vi "Process.vi"(8 "error in":errorcluster, 11 "SynchIO":refnum<class "SynchIO.lvclass">) -> (0 "error out":errorcluster, 3 "SynchIO out":refnum<class "SynchIO.lvclass">)   [LabVIEW 2016, in "SynchIO.lvclass"]
doc: "---------------------------------------------------------------\nJKI State Machine Objects™\nhttp://jki.net/state-machine-objects/\nCopyright (C) 2005-2015, JKI <info@jki.net>\nALL RIGHTS RESERVEDJKI State Machine Objects (SMO) 1.0.0.5\nJKI - JKI\nCopyright (c) 2016, JKI"
uses:
  SynchIO.lvclass
  C:/Program Files (x86)/National Instruments/LabVIEW 2016/vi.lib/JKI/JKI SMO/SMO/SMO.lvclass
  <vilib>/JKI/JKI SMO/SMO/Typedefs/Parent Call--Enum.ctl
  <vilib>/JKI/JKI SMO/SMO/SMO.lvclass
panel:
  # "For instructions on how to use the JKI State Machine Objects, examples and video tutorials, visit:\nhttp://jki.net/state-machine-objects/\n\nJKI State Machine Objects™\nhttp://jki.net/state-machine-objects/\nCopyright (C) 2005-2015, JKI <info@jki.net>\nALL RIGHTS RESERVED"
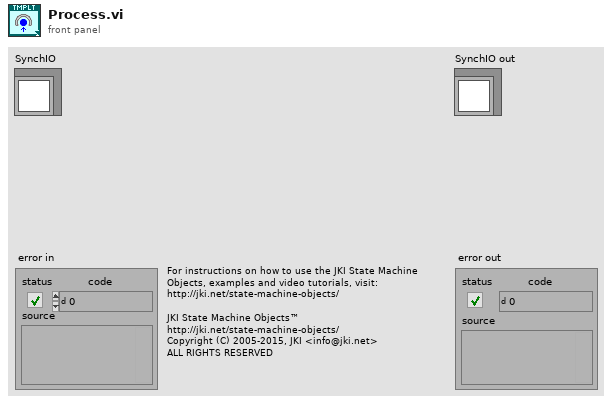
[diagram p1: front panel]
types:
  T1 = typedef "SMO.lvclass/Parent Call--Enum.ctl" = enum16{"Allows parent to run", "Does not request parent to run"}
  T2 = enum32{"invalid app kind", "Development System", "Run Time System", "Student Edition", "Embedded LabVIEW", "Evaluation", "Custom"}
  T3 = enum32{"Invalid", "Standard", "Closed", "Hidden", "Minimized", "Maximized"}
  T4 = cluster{"Core":cluster{"Current VI Reference":refnum<vi>, "Close Panel on Exit?":bool, "error":errorcluster}, "Self Reference":refnum<class "SynchIO.lvclass">, "Your string data":string}
  T5 = cluster{"Current VI Reference":refnum<vi>, "Close Panel on Exit?":bool, "error":errorcluster}
  T6 = typedef "SMO.lvclass/Protected Events.ctl" = cluster{"StopProcesses":refnum<user-event>, "AbortProcesses":refnum<user-event>, "Config Changed":refnum<user-event>, "Dependency":refnum<user-event>}
  T7 = typedef "SynchIO.lvclass/ProtectedEvents--Cluster.ctl" = cluster{"API_Template":refnum<user-event>}
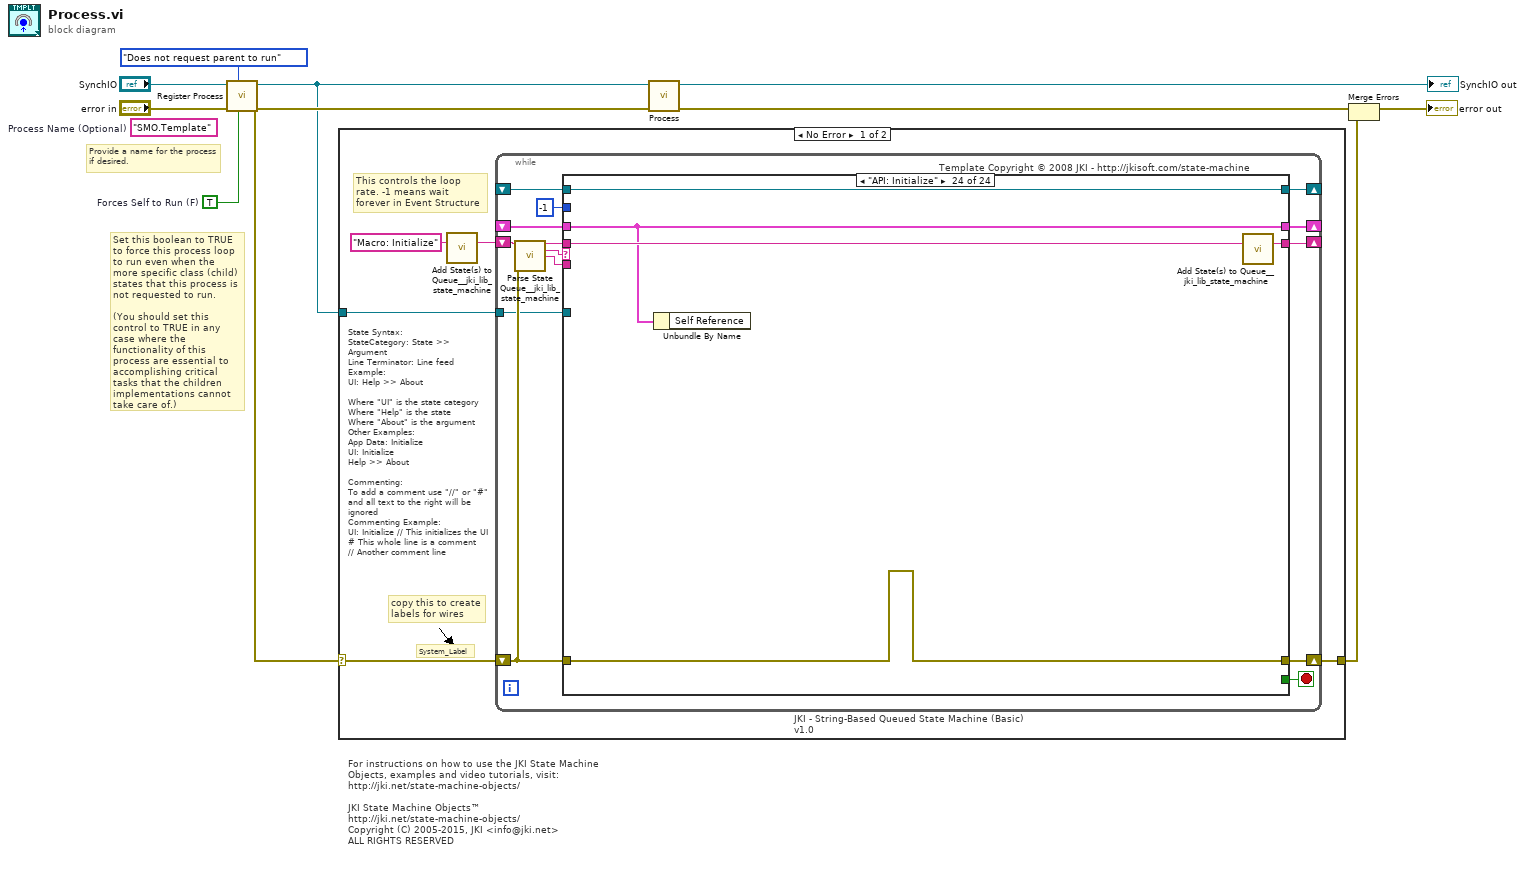
[diagram p0: block diagram]
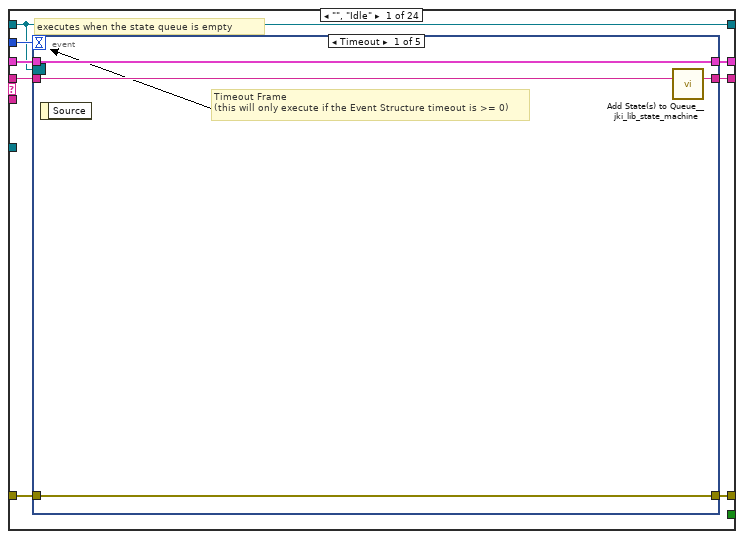
[diagram p2: hidden frame]
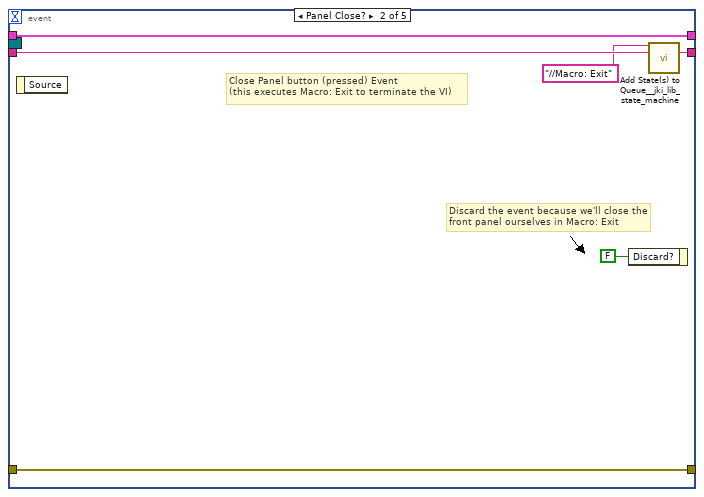
[diagram p3: hidden frame]
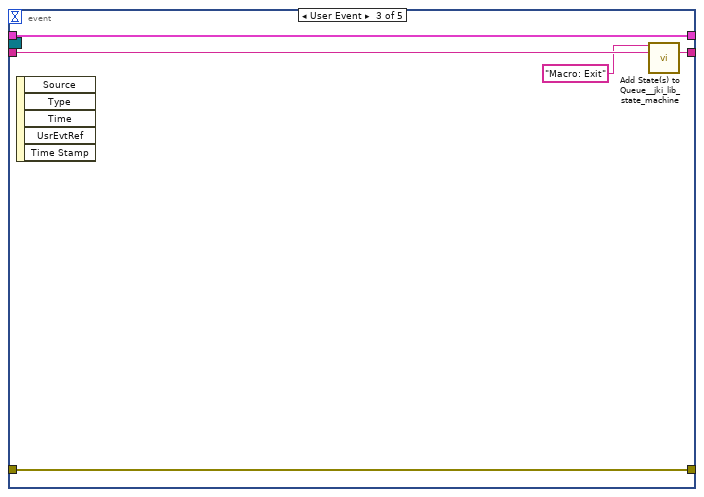
[diagram p4: hidden frame]
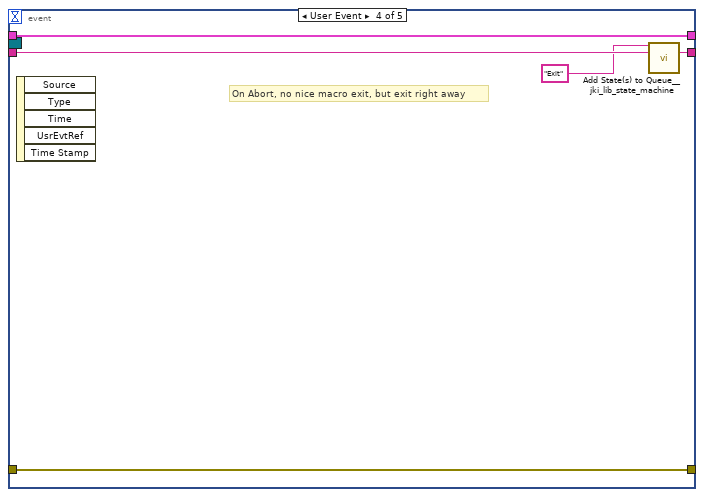
[diagram p5: hidden frame]
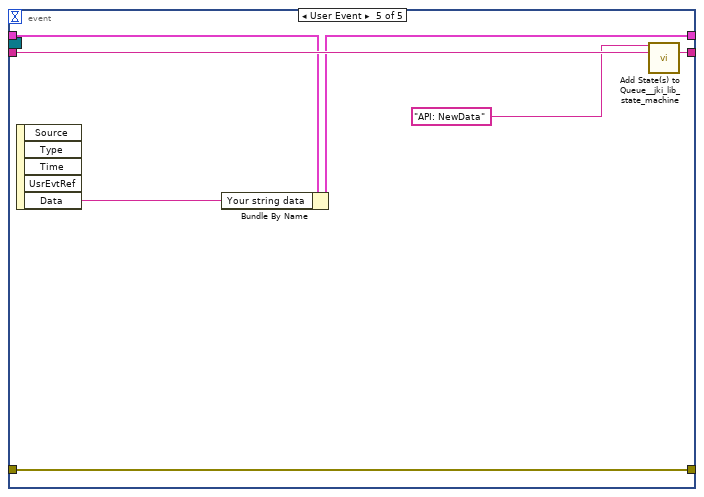
[diagram p6: hidden frame]
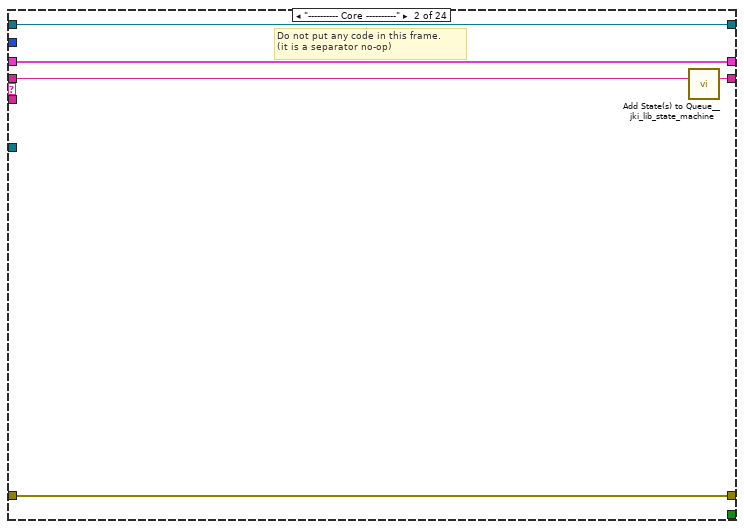
[diagram p7: hidden frame]
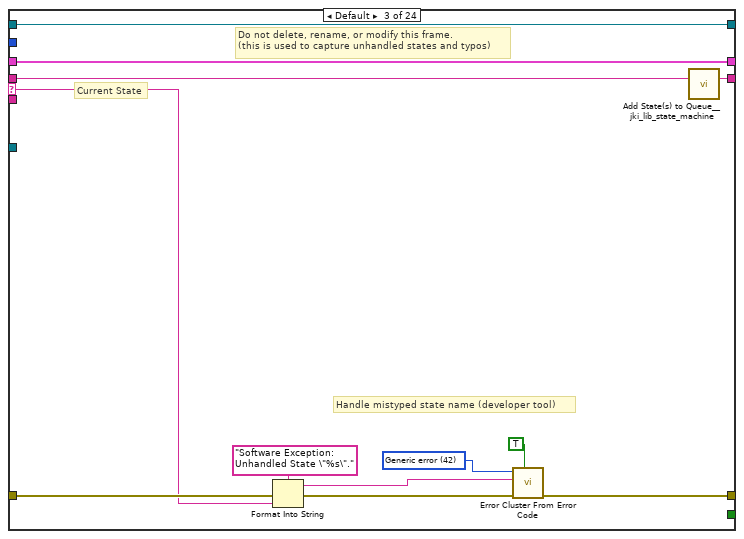
[diagram p8: hidden frame]
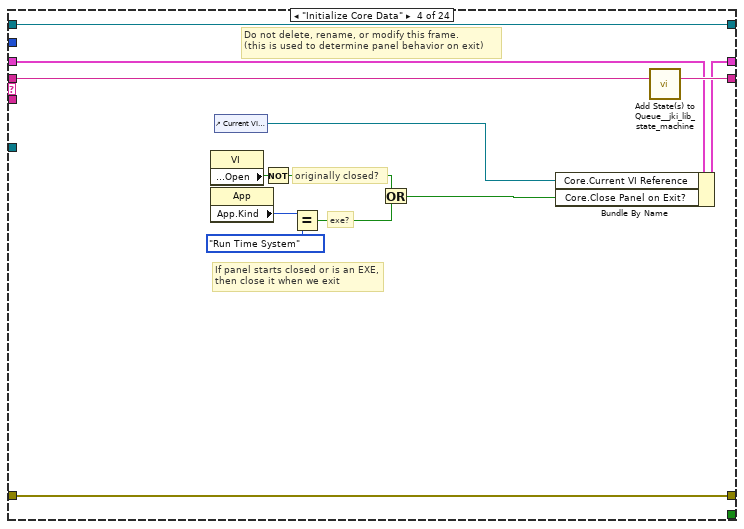
[diagram p9: hidden frame]
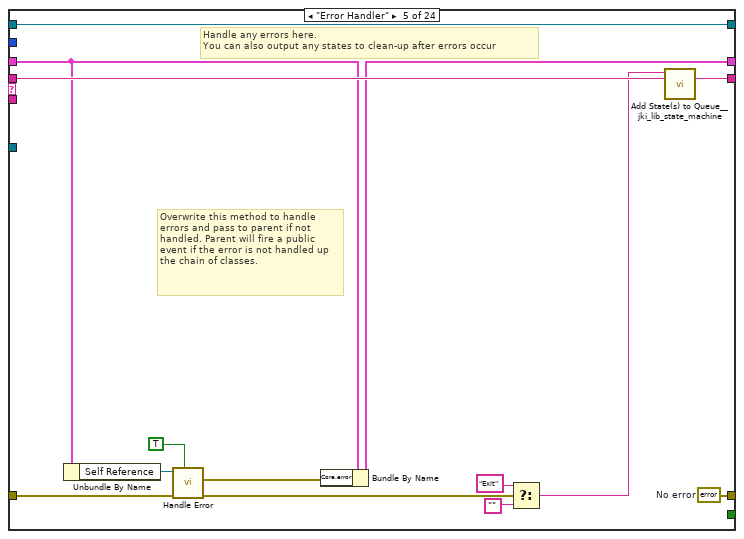
[diagram p10: hidden frame]
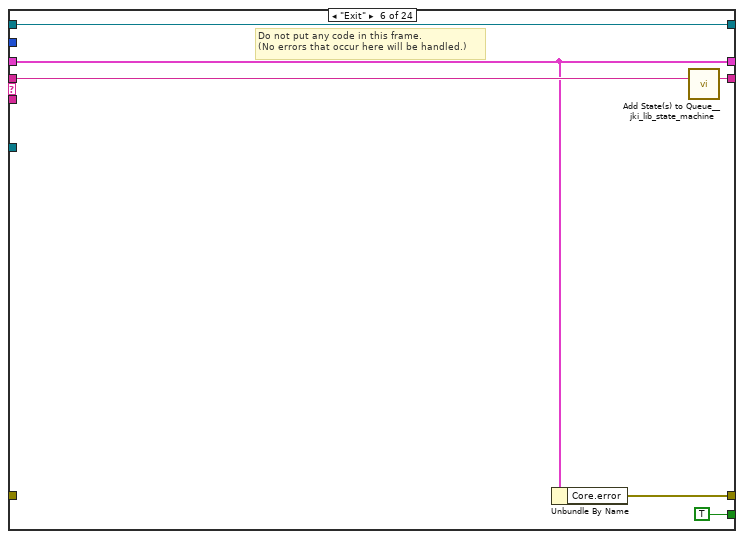
[diagram p11: hidden frame]
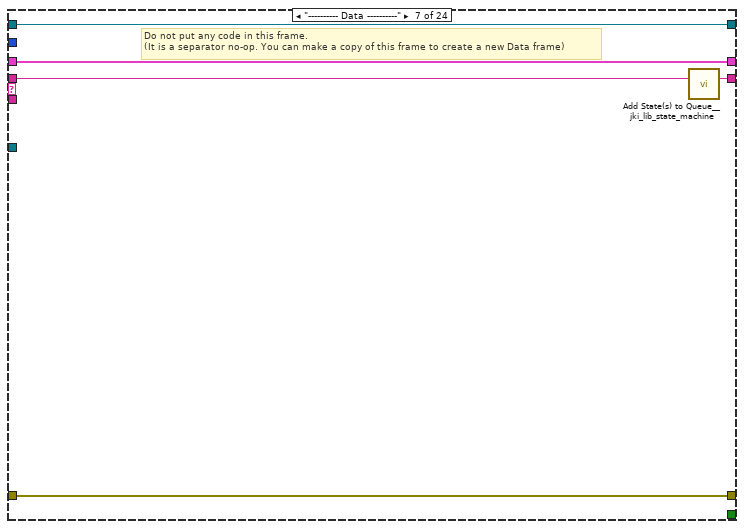
[diagram p12: hidden frame]
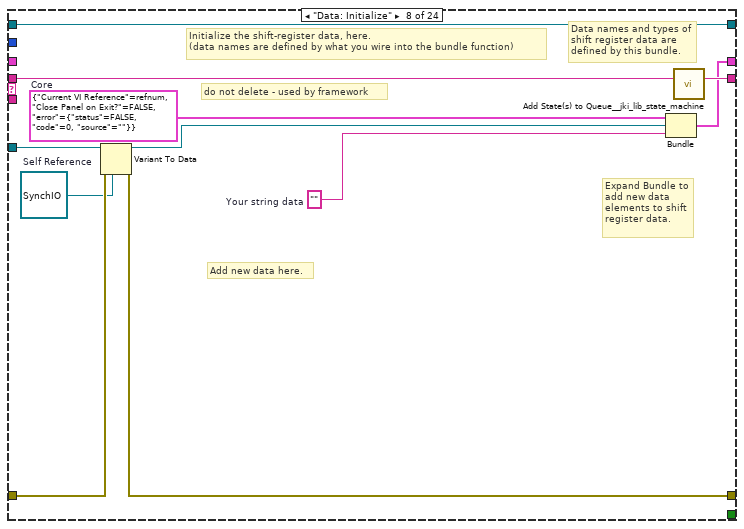
[diagram p13: hidden frame]
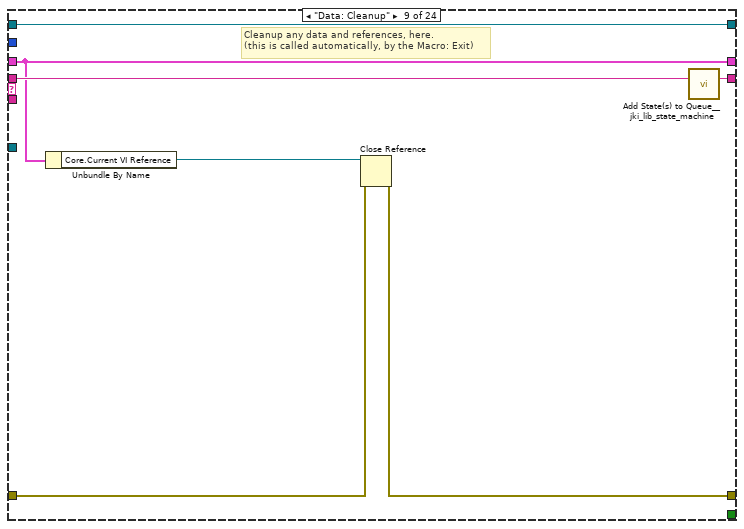
[diagram p14: hidden frame]
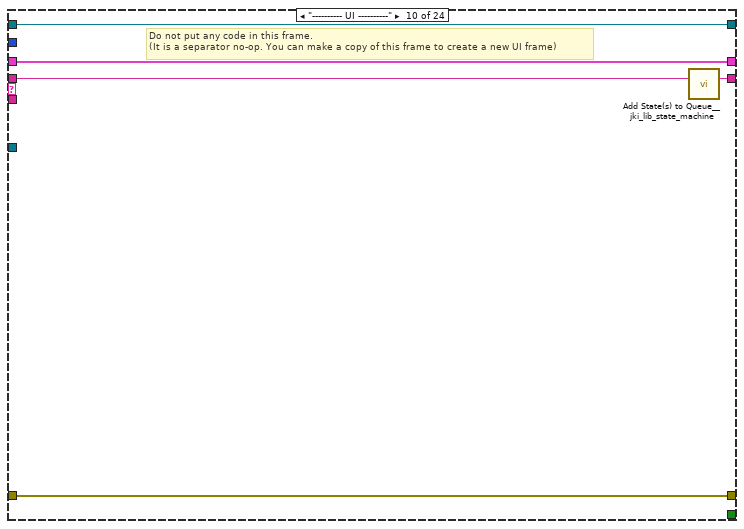
[diagram p15: hidden frame]
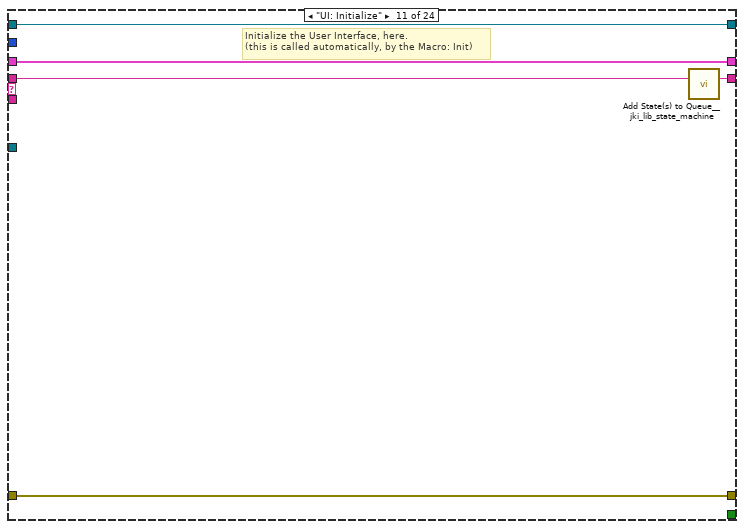
[diagram p16: hidden frame]
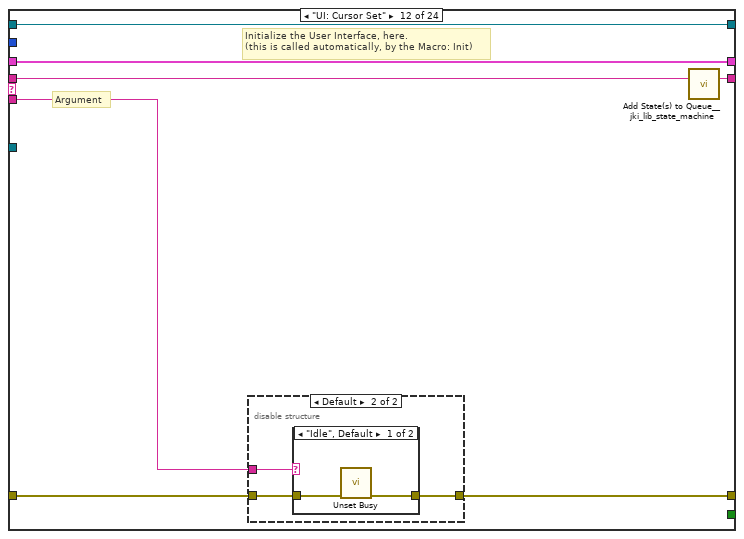
[diagram p17: hidden frame]
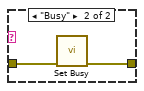
[diagram p19: hidden frame]
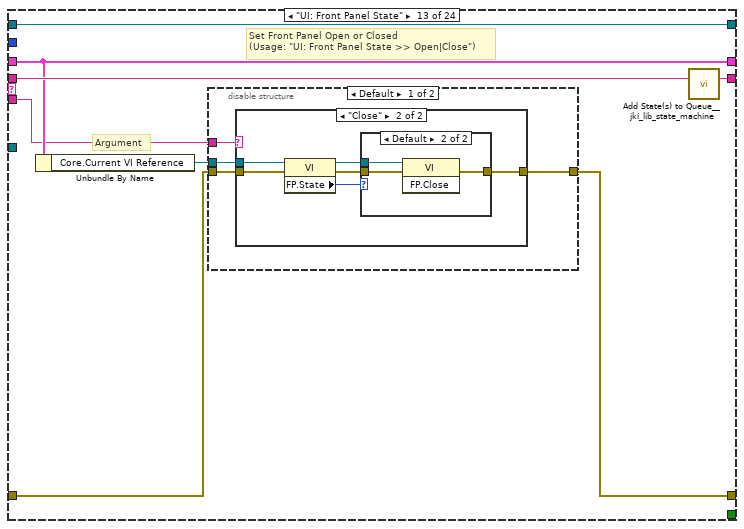
[diagram p20: hidden frame]
diagram:
  w1 = TRUE  # Forces Self to Run (F)
  (unwired) "SMO.Template"  # Process Name (Optional)
  # "Provide a name for the process\nif desired."
  # "Set this boolean to TRUE to force this process loop to run even when the more specific class (child) states that this process is not requested to run.\n\n(You should set this control to TRUE in any case where the functionality of this process are essential to accomplishing critical tasks that the children implementations cannot take care of.)"
  # "For instructions on how to use the JKI State Machine Objects, examples and video tutorials, visit:\nhttp://jki.net/state-machine-objects/\n\nJKI State Machine Objects™\nhttp://jki.net/state-machine-objects/\nCopyright (C) 2005-2015, JKI <info@jki.net>\nALL RIGHTS RESERVED"
  n1 = call <vilib>:"Register Process.vi"("Forces Self to Run (F)"=w1, "Parent Call"=Parent_Call--Enum."Does not request parent to run", "error in (no error)"="error in", "SMO"="SynchIO") -> ("error out"=w7:errorcluster, "SMO out"=w6:refnum<class "SynchIO.lvclass">)  [unwired: 6 in]
  n2 = case shown="No Error" w7 {
    selector: w7 -> [w12 w284]
    tunnel: w6 -> [w13 _]
    tunnel: [w11 w284] -> w3
    frame No Error {
      # "State Syntax:\nStateCategory: State >> Argument\nLine Terminator: Line feed\nExample:\nUI: Help >> About\n\nWhere \"UI\" is the state category\nWhere \"Help\" is the state\nWhere \"About\" is the argument\nOther Examples:\nApp Data: Initialize\nUI: Initialize\nHelp >> About\n\nCommenting:\nTo add a comment use \"//\" or \"#\" and all text to the right will be ignored\nCommenting Example:\nUI: Initialize // This initializes the UI\n# This whole line is a comment\n// Another comment line"
      # "copy this to create labels for wires"
      # "This controls the loop rate. -1 means wait forever in Event Structure"
      # "System_Label"
      n3 = call <vilib>:"Add State(s) to Queue__jki_lib_state_machine.vi"("State(s) in (\"\")"="Macro: Initialize") -> ("States Out"=w15:string)  [unwired: 14 in]
      n4 = while "JKI - String-Based Queued State Machine (Basic) v1.0" {
        shift-right: [w22] -> _
        shift-left: _ -> [w21]
        shift-right: [w25] -> w11
        shift-left: w12 -> [w19]
        shift-right: [w24] -> _
        shift-left: w15 -> [w26]
        tunnel: w13 -> [w18]
        shift-right: [w17] -> _
        shift-left: _ -> [w16]
        stop <- w23 stop-if-true
        # "Template Copyright © 2008 JKI - http://jkisoft.com/state-machine"
        n5 = call <vilib>:"Parse State Queue__jki_lib_state_machine.vi"("State Queue"=w26, "Error In (no error)"=w19) -> ("Remaining States"=w28:string, "Current State"=w29:string, "Arguments"=w27:string)  [unwired: 11 in]
        n6 = case shown="\"API: Initialize\"" w29 {
          selector: w29 -> [_ _ w71 _ _ _ _ _ _ _ _ _ _ _ _ _ _ _ _ _ _ _ _ _]
          tunnel: w28 -> [w37 w69 w75 w94 w108 w114 w119 w130 w137 w142 w147 w154 w170 w202 w211 w225 w230 w241 w246 w259 w265 w270 w278 w283]
          tunnel: w27 -> [_ _ _ _ _ _ _ _ _ _ _ w148 w164 _ _ _ _ _ _ _ _ _ _ _]
          tunnel: w21 -> [w35 w66 w73 w85 w97 w110 w116 _ w132 w139 w145 w152 w166 w199 w207 w216 w227 w238 w243 w257 w263 w268 w275 w280]
          tunnel: [w34 w67 w77 w91 w99 w109 w117 w125 w133 w140 w144 w149 w167 w200 w209 w223 w228 w232 w244 w247 w261 w266 w271 w279] -> w25
          tunnel: w19 -> [w33 w67 w76 w91 w104 _ w117 w126 w134 w140 w144 w150 w168 w200 w209 w223 w228 w233 w244 w251 w261 w266 w272 w279]
          tunnel: [w36 w68 w74 w93 w107 w113 w118 w129 w136 w141 w146 w153 w169 w201 w210 w224 w229 w240 w245 w258 w264 w269 w277 w282] -> w24
          tunnel: [_ _ _ _ _ TRUE _ _ _ _ _ _ _ _ _ _ _ _ _ _ _ _ _ _] -> w23
          tunnel: [w32 w66 w73 w92 w96 w110 w116 w128 w132 w139 w145 w152 w166 w199 w207 w216 w227 w238 w243 w257 w263 w268 w275 w280] -> w22
          tunnel: -1 ("Timeout") -> [w31 _ _ _ _ _ _ _ _ _ _ _ _ _ _ _ _ _ _ _ _ _ _ _]
          tunnel: w18 -> [_ _ _ _ _ _ _ w123 _ _ _ _ _ _ _ _ _ _ _ _ _ _ _ _]
          tunnel: [w30 w65 w70 w82 w106 w111 w115 w121 w131 w138 w143 w151 w163 w198 w208 w217 w226 w239 w242 w256 w262 w267 w276 w281] -> w17
          tunnel: w16 -> [w30 w65 w70 w82 w106 w111 w115 w121 w131 w138 w143 w151 w163 w198 w208 w217 w226 w239 w242 _ w262 w267 w276 w281]
          frame "", "Idle" {
            # "executes when the state queue is empty"
            n7 = event shown="[0] Timeout" {
              selector: w30 -> [_ _ _ _ _]
              dyn-events: _ -> [_ _ _ _ _]
              timeout: w31 -> [_ _ _ _ _]
              tunnel: w37 -> [w41 w47 w52 w57 w64]
              tunnel: [w40 w46 w51 w56 w63] -> w36
              tunnel: w35 -> [w38 w44 w49 w54 w60]
              tunnel: [w39 w45 w50 w55 w62] -> w34
              tunnel: w33 -> [w39 w45 w50 w55 w62]
              tunnel: [w38 w44 w49 w54 w59] -> w32
              event Timeout {
                # "Timeout Frame\n(this will only execute if the Event Structure timeout is >= 0)"
                n8 = event-data() -> ()  [unwired: 1 in, 1 out]
                n9 = call <vilib>:"Add State(s) to Queue__jki_lib_state_machine.vi"("State(s) in (\"\")"=w41) -> ("States Out"=w40:string)  [unwired: 14 in]
              }
              event Panel Close? {
                # "Discard the event because we'll close the front panel ourselves in Macro: Exit"
                # "Close Panel button (pressed) Event\n(this executes Macro: Exit to terminate the VI)"
                n10 = event-data() -> ()  [unwired: 1 in, 1 out]
                n11 = event-data("Discard?"=FALSE) -> ()  [unwired: 1 in, 1 out]
                n12 = call <vilib>:"Add State(s) to Queue__jki_lib_state_machine.vi"("State(s) in Front (\"\")"="//Macro: Exit", "State(s) in (\"\")"=w47) -> ("States Out"=w46:string)  [unwired: 13 in]
              }
              event User Event {
                n13 = event-data() -> ()  [unwired: 1 in, 5 out]
                n14 = call <vilib>:"Add State(s) to Queue__jki_lib_state_machine.vi"("State(s) in Front (\"\")"="Macro: Exit", "State(s) in (\"\")"=w52) -> ("States Out"=w51:string)  [unwired: 13 in]
              }
              event User Event {
                # "On Abort, no nice macro exit, but exit right away"
                n15 = event-data() -> ()  [unwired: 1 in, 5 out]
                n16 = call <vilib>:"Add State(s) to Queue__jki_lib_state_machine.vi"("State(s) in Front (\"\")"="Exit", "State(s) in (\"\")"=w57) -> ("States Out"=w56:string)  [unwired: 13 in]
              }
              event User Event {
                n17 = event-data() -> ("Data"=w61:string)  [unwired: 1 in, 4 out]
                n18 = Bundle By Name(cluster=w60, "Your string data"=w61) -> (w59:T4)
                n19 = call <vilib>:"Add State(s) to Queue__jki_lib_state_machine.vi"("State(s) in Front (\"\")"="API: NewData", "State(s) in (\"\")"=w64) -> ("States Out"=w63:string)  [unwired: 13 in]
              }
            }
          }
          frame "---------- Core ----------" {
            # "Do not put any code in this frame.\n(it is a separator no-op)"
            n20 = call <vilib>:"Add State(s) to Queue__jki_lib_state_machine.vi"("State(s) in (\"\")"=w69) -> ("States Out"=w68:string)  [unwired: 14 in]
          }
          frame Default {
            w80 = 42 items=["No error", "Argument error", "Memory is full", "Out of zone", "End of file", "File already open", "Generic file I/O error", "File not found", "File permission error", "Disk is full", "Duplicate path", "Too many files open", "System feature not enabled", "Resource file not found", "Cannot add resource", "Resource not found", "Image not found", "Image memory error", "Pen does not exist", "Config type invalid", "Config token not found", "Config parse error", "Config memory error", "Bad external code format", "Bad external code offset", "External code not present", "Null window", "Destroy window error", "Null menu", "Print aborted", "Bad print record", "Print driver error", "Windows error during printing", "Memory error during printing", "Print dialog error", "Generic print error", "Invalid device refnum", "Device not found", "Device parameter error", "Device unit error", "Cannot open device", "Device call aborted", "Generic error", "Cancelled by user", "Object ID too low", "Object ID too high", "Object not in heap", "Unknown heap", "Unknown object (invalid DefProc)", "Unknown object (DefProc not in table)", "Message out of range", "Invalid (null) method", "Unknown message", "Manager call not supported", "Bad address", "Network operation in progress", "Network operation timed out", "Connection is busy", "Network attribute not supported", "Network error", "Address in use", "System out of memory", "Connection aborted", "Connection refused", "Not connected", "Already connected", "Connection closed", "Initialization error (interapplication manager)", "Bad occurrence", "Wait on unbound occurrence handler", "Occurrence queue overflow", "Datalog type conflict", "Unused", "Unrecognized type (interapplication manager)", "Memory corrupt", "Failed to make temporary DLL", "Old CIN version", "Drag socket not found", "Failed to load drop-object", "Failed to register OLE object", "Failed to release OLE object", "Format specifier type mismatch", "Unknown format specifier", "Too few format specifiers", "Too many format specifiers", "Scan failed", "Newer CIN version", "Error converting to variant", "Runtime menu error", "Password tampered", "Variant attribute not found", "Incompatible variant data type", "Event data is not available", "Event Store is not present", "Occurrence is not found", "Event Queue is not created", "Event info is not available", "Refnum passed is NULL", "Error retrieving Class GUID", "Error retrieving CoClass GUID", "Error retrieving TypeLib GUID.", "Bad built application magic bytes.", "Specific driver is different from the specific driver associated with the Logical Name.", "There is no session opened to the class driver.", "Max Error", "MAX - Error with config objects", "MAX - Error loading configuration", "MAX - Group not supported"]
            # "Current State"
            # "Do not delete, rename, or modify this frame.\n(this is used to capture unhandled states and typos)"
            # "Handle mistyped state name (developer tool)"
            n21 = Format Into String(format string="Software Exception: Unhandled State \"%s\"." ("message"), error in=w76, w71) -> (resulting string=w79:string, error out=w78:errorcluster)  [unwired: 1 in]
            n22 = call <vilib>:"Error Cluster From Error Code.vi"("show call chain? (False)"=TRUE, "error in (no error)"=w78, "error message (\"\")"=w79, "error code (0)"=w80) -> ("error out"=w77:errorcluster)  [unwired: 5 in]
            n23 = call <vilib>:"Add State(s) to Queue__jki_lib_state_machine.vi"("State(s) in (\"\")"=w75) -> ("States Out"=w74:string)  [unwired: 14 in]
          }
          frame "Initialize Core Data" {
            # "Do not delete, rename, or modify this frame.\n(this is used to determine panel behavior on exit)"
            # "originally closed?"
            # "exe?"
            # "If panel starts closed or is an EXE, then close it when we exit"
            n24 = property class="VI"() -> ("Front Panel.Open"=w90:bool)  [unwired: 2 in, 2 out]
            n25 = property class="App"() -> ("App.Kind"=w89:T2)  [unwired: 2 in, 2 out]
            n26 = control-ref of="Current VI Reference"() -> (w83:refnum<vi>)
            n27 = Not(x=w90) -> (.not. x?=w87:bool)
            n28 = Equal?(x=w89, y=T2."Run Time System" ("Application:Kind")) -> (x = y?=w86:bool)
            n29 = Or(x=w87, y=w86) -> (x .or. y?=w84:bool)
            n30 = Bundle By Name(cluster=w85, "Core.Current VI Reference"=w83, "Core.Close Panel on Exit?"=w84) -> (w92:T4)
            n31 = call <vilib>:"Add State(s) to Queue__jki_lib_state_machine.vi"("State(s) in (\"\")"=w94) -> ("States Out"=w93:string)  [unwired: 14 in]
          }
          frame "Error Handler" {
            w99 = errorcluster {"status"=FALSE, "code"=0, "source"=""}  # No error
            # "Overwrite this method to handle errors and pass to parent if not handled. Parent will fire a public event if the error is not handled up the chain of classes."
            # "Handle any errors here.\nYou can also output any states to clean-up after errors occur"
            n32 = Unbundle By Name(w97) -> ("Self Reference"=w105:refnum<class "SynchIO.lvclass">)
            n33 = call-dynamic "Handle Error.vi"("Stop on Unhandled Error (T)"=TRUE, "error in"=w104, "SMO"=w105) -> ("handling error"=w100:errorcluster, "Unhandled error"=w98:errorcluster)  [unwired: 6 in, 1 out]
            n34 = Bundle By Name(cluster=w97, "Core.error"=w98) -> (w96:T4)
            n35 = Select(t="Exit", s=w100, f="") -> (s? t:f=w101:string)
            n36 = call <vilib>:"Add State(s) to Queue__jki_lib_state_machine.vi"("State(s) in Front (\"\")"=w101, "State(s) in (\"\")"=w108) -> ("States Out"=w107:string)  [unwired: 13 in]
          }
          frame "Exit" {
            # "Do not put any code in this frame.\n(No errors that occur here will be handled.)"
            n37 = Unbundle By Name(w110) -> ("Core.error"=w109:errorcluster)
            n38 = call <vilib>:"Add State(s) to Queue__jki_lib_state_machine.vi"("State(s) in (\"\")"=w114) -> ("States Out"=w113:string)  [unwired: 14 in]
          }
          frame "---------- Data ----------" {
            # "Do not put any code in this frame.\n(It is a separator no-op. You can make a copy of this frame to create a new Data frame)"
            n39 = call <vilib>:"Add State(s) to Queue__jki_lib_state_machine.vi"("State(s) in (\"\")"=w119) -> ("States Out"=w118:string)  [unwired: 14 in]
          }
          frame "Data: Initialize" {
            w120 = T5 {"Current VI Reference"=refnum, "Close Panel on Exit?"=FALSE, "error"={"status"=FALSE, "code"=0, "source"=""}}  # Core
            w124 = refnum<class "SynchIO.lvclass"> refnum  # Self Reference
            w127 = ""  # Your string data
            # "do not delete - used by framework"
            # "Expand Bundle to add new data elements to shift register data."
            # "Add new data here."
            # "Data names and types of shift register data are defined by this bundle."
            # "Initialize the shift-register data, here.\n(data names are defined by what you wire into the bundle function)"
            n40 = Variant To Data(error in=w126, type=w124, Variant=w123) -> (data=w122:refnum<class "SynchIO.lvclass">, error out=w125:errorcluster)
            n41 = Bundle("Core"=w120, "Self Reference"=w122, "Your string data"=w127) -> (w128:T4)  [unwired: 1 in]
            n42 = call <vilib>:"Add State(s) to Queue__jki_lib_state_machine.vi"("State(s) in (\"\")"=w130) -> ("States Out"=w129:string)  [unwired: 14 in]
          }
          frame "Data: Cleanup" {
            # "Cleanup any data and references, here.\n(this is called automatically, by the Macro: Exit)"
            n43 = Unbundle By Name(w132) -> ("Core.Current VI Reference"=w135:refnum<vi>)
            n44 = Close Reference(reference=w135, error in (no error)=w134) -> (error out=w133:errorcluster)
            n45 = call <vilib>:"Add State(s) to Queue__jki_lib_state_machine.vi"("State(s) in (\"\")"=w137) -> ("States Out"=w136:string)  [unwired: 14 in]
          }
          frame "---------- UI ----------" {
            # "Do not put any code in this frame.\n(It is a separator no-op. You can make a copy of this frame to create a new UI frame)"
            n46 = call <vilib>:"Add State(s) to Queue__jki_lib_state_machine.vi"("State(s) in (\"\")"=w142) -> ("States Out"=w141:string)  [unwired: 14 in]
          }
          frame "UI: Initialize" {
            # "Initialize the User Interface, here.\n(this is called automatically, by the Macro: Init)"
            n47 = call <vilib>:"Add State(s) to Queue__jki_lib_state_machine.vi"("State(s) in (\"\")"=w147) -> ("States Out"=w146:string)  [unwired: 14 in]
          }
          frame "UI: Cursor Set" {
            # "Argument"
            # "Initialize the User Interface, here.\n(this is called automatically, by the Macro: Init)"
            n48 = disable-structure shown="Default" {
              disable-tunnel: w150 -> [w155 w158]
              disable-tunnel: [w155 w157] -> w149
              disable-tunnel: w148 -> [_ w156]
              frame condition #0 {
              }
              frame condition #1 (active) {
                n49 = case shown="\"Idle\", Default" w156 {
                  tunnel: w158 -> [w160 w162]
                  tunnel: [w159 w161] -> w157
                  frame "Idle", Default {
                    n50 = call <vilib>:"Unset Busy.vi"("error in (no error)"=w160) -> ("error out"=w159:errorcluster)  [unwired: 10 in]
                  }
                  frame "Busy" {
                    n51 = call <vilib>:"Set Busy.vi"("error in (no error)"=w162) -> ("error out"=w161:errorcluster)  [unwired: 9 in, 1 out]
                  }
                }
              }
            }
            n52 = call <vilib>:"Add State(s) to Queue__jki_lib_state_machine.vi"("State(s) in (\"\")"=w154) -> ("States Out"=w153:string)  [unwired: 14 in]
          }
          frame "UI: Front Panel State" {
            # "Argument"
            # "Set Front Panel Open or Closed\n(Usage: \"UI: Front Panel State >> Open|Close\")"
            n53 = Unbundle By Name(w166) -> ("Core.Current VI Reference"=w165:refnum<vi>)
            n54 = disable-structure shown="Default" {
              disable-tunnel: w168 -> [w174 w197]
              disable-tunnel: [w173 w197] -> w167
              disable-tunnel: w165 -> [w172 _]
              disable-tunnel: w164 -> [w171 _]
              frame condition #0 (active) {
                n55 = case shown="\"Close\"" w171 {
                  tunnel: w174 -> [w178 w191]
                  tunnel: [w180 w192] -> w173
                  tunnel: w172 -> [w179 w189]
                  frame "Open", Default {
                    n56 = property class="VI"(reference=w179, error in=w178) -> (reference out=w176:refnum<vi>, error out=w177:errorcluster, "FP.State"=w175:T3)
                    n57 = case shown="\"Closed\"" w175 {
                      tunnel: [w183 w186] -> w180
                      tunnel: w177 -> [w182 w186]
                      tunnel: w176 -> [w181 _]
                      frame "Closed" {
                        n58 = invoke class="VI" method="FP.Open"(reference=w181, error in=w182, "Activate"=TRUE, "State"=T3."Standard") -> (error out=w183:errorcluster)  [unwired: 1 in, 4 out]
                      }
                      frame Default {
                      }
                    }
                  }
                  frame "Close" {
                    n59 = property class="VI"(reference=w189, error in=w191) -> (reference out=w188:refnum<vi>, error out=w190:errorcluster, "FP.State"=w187:T3)
                    n60 = case shown="Default" w187 {
                      tunnel: [w193 w196] -> w192
                      tunnel: w190 -> [w193 w195]
                      tunnel: w188 -> [_ w194]
                      frame "Invalid", "Closed" {
                      }
                      frame Default {
                        n61 = invoke class="VI" method="FP.Close"(reference=w194, error in=w195) -> (error out=w196:errorcluster)  [unwired: 1 in, 2 out]
                      }
                    }
                  }
                }
              }
              frame condition #1 {
              }
            }
            n62 = call <vilib>:"Add State(s) to Queue__jki_lib_state_machine.vi"("State(s) in (\"\")"=w170) -> ("States Out"=w169:string)  [unwired: 14 in]
          }
          frame "---------- Macro ----------" {
            # "Do not put any code in this frame.\n(It is a separator no-op. You can make a copy of this frame to create a new Macro frame)"
            n63 = call <vilib>:"Add State(s) to Queue__jki_lib_state_machine.vi"("State(s) in (\"\")"=w202) -> ("States Out"=w201:string)  [unwired: 14 in]
          }
          frame "Macro: Initialize" {
            w205 = "UI: Initialize\n//UI: Front Panel State >> Open"  # UI: Initialize //UI: Front Panel State >> Open
            # "Initialization Macro\n(This is called once, when the VI starts)"
            n64 = call <vilib>:"Add State(s) to Queue__jki_lib_state_machine.vi"("State(s) in Front (\"\")"="Data: Initialize\nInitialize Core Data\nEvents: Register", "State(s) in (\"\")"="Process: Sync", "State(s) at Back (\"\")"=w205) -> ("States Out"=w204:string)  [unwired: 12 in]
            n65 = call <vilib>:"Add State(s) to Queue__jki_lib_state_machine.vi"("State(s) in Front (\"\")"=w204, "State(s) in (\"\")"=w211) -> ("States Out"=w210:string)  [unwired: 13 in]
          }
          frame "Macro: Exit" {
            # "Exit Macro\n(This is called once, when the VI exits)"
            n66 = Unbundle By Name(w216) -> ("Core.Close Panel on Exit?"=w222:bool)
            n67 = Select(t="UI: Front Panel State >> Close", s=w222, f="") -> (s? t:f=w219:string)
            n68 = call <vilib>:"Add State(s) to Queue__jki_lib_state_machine.vi"("State(s) in Front (\"\")"="Data: Cleanup\nEvents: Unregister", "State(s) in (\"\")"="Process: Sync", "State(s) at Back (\"\")"="Exit") -> ("States Out"=w213:string)  [unwired: 12 in]
            n69 = call <vilib>:"Add State(s) to Queue__jki_lib_state_machine.vi"("State(s) in (\"\")"=w219, "State(s) at Back (\"\")"=w213) -> ("States Out"=w218:string)  [unwired: 13 in]
            n70 = call <vilib>:"Add State(s) to Queue__jki_lib_state_machine.vi"("State(s) in Front (\"\")"=w218, "State(s) in (\"\")"=w225) -> ("States Out"=w224:string)  [unwired: 13 in]
          }
          frame "---------- Process ----------" {
            # "Template Separator\n(You can make a copy of, or modify, this frame)"
            n71 = call <vilib>:"Add State(s) to Queue__jki_lib_state_machine.vi"("State(s) in (\"\")"=w230) -> ("States Out"=w229:string)  [unwired: 14 in]
          }
          frame "Process: Sync" {
            n72 = Unbundle By Name(w238) -> ("Self Reference"=w234:refnum<class "SynchIO.lvclass">)
            n73 = call <vilib>:"WaitOnProcessSync.vi"("error in (no error)"=w233, "SMO"=w234) -> ("error out"=w232:errorcluster, "Don't run?"=w237:bool)  [unwired: 7 in, 1 out]
            n74 = Select(t="Data: Cleanup\nEvents: Unregister\nExit", s=w237, f="") -> (s? t:f=w231:string)
            n75 = call <vilib>:"Add State(s) to Queue__jki_lib_state_machine.vi"("State(s) in Front (\"\")"=w231, "State(s) in (\"\")"=w241) -> ("States Out"=w240:string)  [unwired: 13 in]
          }
          frame "---------- Events ----------" {
            # "Template Separator\n(You can make a copy of, or modify, this frame)"
            n76 = call <vilib>:"Add State(s) to Queue__jki_lib_state_machine.vi"("State(s) in (\"\")"=w246) -> ("States Out"=w245:string)  [unwired: 14 in]
          }
          frame "Events: Register" {
            # "Expand to add\nmore events"
            # "Self Events (API Calls)"
            # "Base Class Protected Events"
            n77 = Unbundle By Name(w257) -> ("Self Reference"=w252:refnum<class "SynchIO.lvclass">)
            n78 = call <vilib>:"GetProtectedEvents.vi"("SMO"=w252) -> ("error out"=w248:errorcluster, "SMO Protected Events"=w255:T6, "SMO out"=w254:refnum<class "SynchIO.lvclass">)  [unwired: 8 in]
            n79 = call "SynchIO.GetProtectedEvents.vi"("SynchIO"=w254) -> ("error out"=w249:errorcluster, "Protected Events"=w253:T7)  [unwired: 8 in, 1 out]
            n80 = register-events(w255, w253) -> (reference out=w256:refnum<event-registration>, error out=w250:errorcluster)  [unwired: 2 in]
            n81 = Merge Errors(w251, w250, w249, w248) -> (w247:errorcluster)
            n82 = call <vilib>:"Add State(s) to Queue__jki_lib_state_machine.vi"("State(s) in (\"\")"=w259) -> ("States Out"=w258:string)  [unwired: 14 in]
          }
          frame "Events: Unregister" {
            n83 = Unregister For Events(event registration refnum=w262, error in=w261) -> (error out=w260:errorcluster)
            n84 = call <vilib>:"Clear Errors.vi"("error in (no error)"=w260) -> ()  [unwired: 5 in, 2 out]
            n85 = call <vilib>:"Add State(s) to Queue__jki_lib_state_machine.vi"("State(s) in (\"\")"=w265) -> ("States Out"=w264:string)  [unwired: 14 in]
          }
          frame "---------- API ----------" {
            n86 = call <vilib>:"Add State(s) to Queue__jki_lib_state_machine.vi"("State(s) in (\"\")"=w270) -> ("States Out"=w269:string)  [unwired: 14 in]
          }
          frame "API: NewData" {
            n87 = Unbundle By Name(w275) -> ("Self Reference"=w274:refnum<class "SynchIO.lvclass">, "Your string data"=w273:string)
            n88 = call "SynchIO.SetData.vi"("error in (no error)"=w272, "Data In"=w273, "SynchIO"=w274) -> ("error out"=w271:errorcluster)  [unwired: 7 in, 1 out]
            n89 = call <vilib>:"Add State(s) to Queue__jki_lib_state_machine.vi"("State(s) in (\"\")"=w278) -> ("States Out"=w277:string)  [unwired: 14 in]
          }
          frame "API: Initialize" {
            n90 = Unbundle By Name(w280) -> ()  [unwired: 1 out]
            n91 = call <vilib>:"Add State(s) to Queue__jki_lib_state_machine.vi"("State(s) in (\"\")"=w283) -> ("States Out"=w282:string)  [unwired: 14 in]
          }
        }
      }
    }
    frame Error {
    }
  }
  n92 = call-parent "Process.vi"("error in"=w7, "SMO"=w6) -> ("error out"=w4:errorcluster, "SMO out"=→"SynchIO out":refnum<class "SynchIO.lvclass">)  [unwired: 8 in]
  n93 = Merge Errors(w4, w3) -> (→"error out":errorcluster)
